vi "Set Ramping Mode_brasse.vi"(1 "error in":T2, 2 "Ramping Mode":u16(ring) items=["RAMP", "PAUSE", "MANUAL UP", "MANUAL DOWN", "ZERO"], 3 "Communications Config":T1={"GPIB address"=22, "GPIB bus"=0, "connection ID"=refnum, "IP"="192.168.2.200", "Active Comm Interface"=0, "Serial Port"="", "Programmer Type"=0} {"Programmer Type" items=["Model 430", "Model 420"]; "Active Comm Interface" items=["TCP/IP (Model 430 Only)", "RS232", "IEEE488"]}) -> (0 "error out":T2)   [LabVIEW 2009]
panel:
  in  "GPIB Address":cluster{"GPIB address":i16, "GPIB bus":i16}={"GPIB address"=22, "GPIB bus"=0}
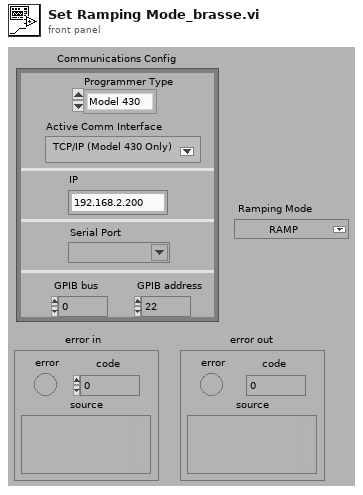
[diagram p1: front panel]
types:
  T1 = cluster{"GPIB address":i16, "GPIB bus":i16, "connection ID":refnum<k5>, "IP":string, "Active Comm Interface":u16, "Serial Port":refnum<visa-resource-name>, "Programmer Type":u16}
  T2 = cluster{"error":bool, "code":i32, "source":string}
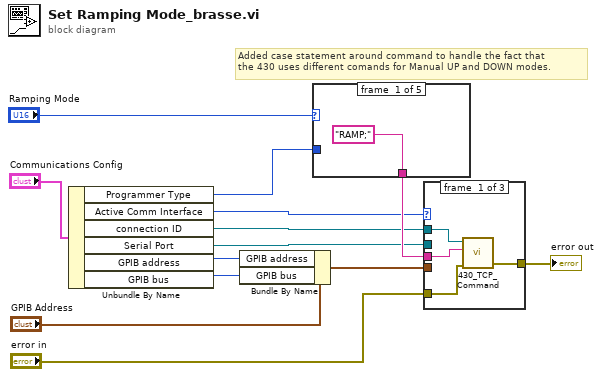
[diagram p0: block diagram]
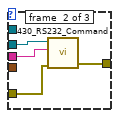
[diagram p2: hidden frame]
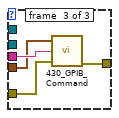
[diagram p3: hidden frame]
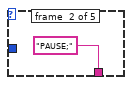
[diagram p4: hidden frame]
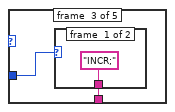
[diagram p5: hidden frame]
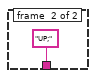
[diagram p6: hidden frame]
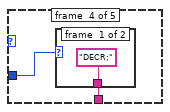
[diagram p7: hidden frame]
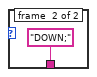
[diagram p8: hidden frame]
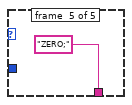
[diagram p9: hidden frame]
diagram:
  # "Added case statement around command to handle the fact that\nthe 430 uses different comands for Manual UP and DOWN modes."
  n1 = Unbundle By Name("Communications Config") -> ("Programmer Type"=w1:u16, "Active Comm Interface"=w2:u16, "connection ID"=w8:refnum<k5>, "Serial Port"=w7:refnum<visa-resource-name>, "GPIB address"=w11:i16, "GPIB bus"=w10:i16)
  n2 = Bundle By Name(cluster="GPIB Address", "GPIB address"=w11, "GPIB bus"=w10) -> (w6:cluster{"GPIB address":i16, "GPIB bus":i16})
  n3 = case shown="2" "Ramping Mode" {
    tunnel: w1 -> [_ _ w17 w21 _]
    tunnel: ["RAMP;" "PAUSE;" w16 w20 "ZERO;"] -> w9
    frame #0 {
    }
    frame #1 {
    }
    frame #2 {
      n4 = case shown="1" w17 {
        tunnel: ["INCR;" "UP;"] -> w16
        frame #0 {
        }
        frame #1 {
        }
      }
    }
    frame #3 {
      n5 = case shown="1" w21 {
        tunnel: ["DECR;" "DOWN;"] -> w20
        frame #0 {
        }
        frame #1 {
        }
      }
    }
    frame #4 {
    }
  }
  n6 = case shown="2" w2 {
    tunnel: w7 -> [_ w29 _]
    tunnel: "error in" -> [w27 w31 w36]
    tunnel: w9 -> [w26 w30 w35]
    tunnel: [w28 w32 w34] -> w4
    tunnel: w8 -> [w25 _ _]
    tunnel: w6 -> [_ _ w33]
    frame #0 {
      n7 = call <userlib>:"430_TCP_Command.vi"("error in (no error)"=w27, "Command"=w26, "connection ID"=w25) -> ("error out"=w28:errorcluster)  [unwired: 1 in, 2 out]
    }
    frame #1 {
      n8 = call <userlib>:"430_RS232_Command.vi"("error in (no error)"=w31, "Command"=w30, "VISA resource name"=w29) -> ("error out"=w32:errorcluster)  [unwired: 1 in, 2 out]
    }
    frame #2 {
      n9 = call <userlib>:"430_GPIB_Command.vi"("GPIB (In)"=w33, "Input command"=w35, "error in"=w36) -> ("error out"=w34:T2)  [unwired: 3 out]
    }
  }
  "error out" <- w4
